vi "is_page.vi"(1 "ctrl ref":refnum<vi>) -> (0 "is page?":bool)   [LabVIEW 2015]
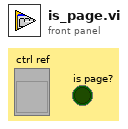
[diagram p1: front panel]
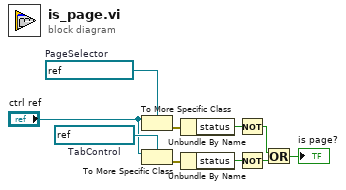
[diagram p0: block diagram]
diagram:
  w7 = refnum<vi> refnum  # PageSelector
  w8 = refnum<vi> refnum  # TabControl
  n1 = To More Specific Class(target class=w7, reference="ctrl ref") -> (error out=w4:errorcluster)  [unwired: 1 in, 1 out]
  n2 = To More Specific Class(target class=w8, reference="ctrl ref") -> (error out=w10:errorcluster)  [unwired: 1 in, 1 out]
  n3 = Unbundle By Name(w4) -> ("status"=w5:bool)
  n4 = Unbundle By Name(w10) -> ("status"=w9:bool)
  n5 = Not(x=w5) -> (.not. x?=w3:bool)
  n6 = Not(x=w9) -> (.not. x?=w2:bool)
  n7 = Or(x=w3, y=w2) -> (x .or. y?=→"is page?":bool)
